vi "Error Handler - Message Handling Loop.vi"(8 "error in (no error)":errorcluster, 10 "Ignore Errors (Runtime)":i32[](array[numeric]), 11 "Message Queue":refnum<queue>) -> (0 "dup error in":errorcluster, 3 "dup Message Queue":refnum<queue>)   [LabVIEW 2017]
doc: "Process an error that occurred in the Message Handling Loop, either by ignoring it, or generating an \"Exit\" message."
uses:
  Message Queue/Message Cluster.ctl
  Message Queue/Message Queue.lvlib
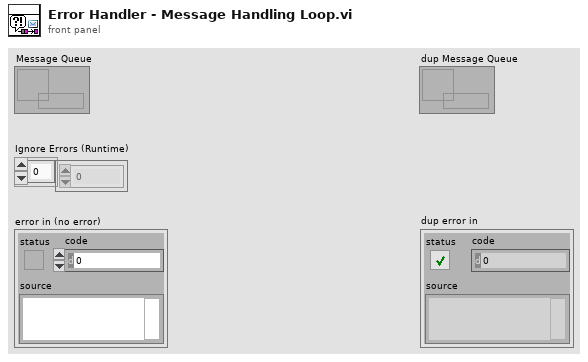
[diagram p1: front panel]
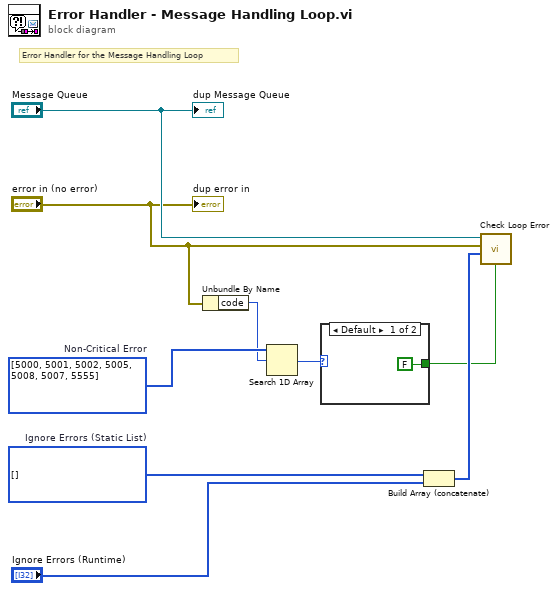
[diagram p0: block diagram]
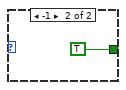
[diagram p2: hidden frame]
diagram:
  w3 = i32[] [5000, 5001, 5002, 5005, 5008, 5007, 5555]  # Non-Critical Error
  w8 = i32[] []  # Ignore Errors (Static List)
  # "Error Handler for the Message Handling Loop"
  n1 = Unbundle By Name("error in (no error)") -> ("code"=w2:i32)
  n2 = Search 1D Array(1D array=w3, element=w2) -> (index of element=w1:i32)  [unwired: 1 in]
  n3 = case shown="Default" w1 {
    tunnel: [FALSE ("Exit on Error? (F)") TRUE ("Exit on Error? (F)")] -> w5
    frame Default {
    }
    frame -1 {
    }
  }
  n4 = Build Array (concatenate)(w8, "Ignore Errors (Runtime)") -> (w7:i32[])
  n5 = call "Check Loop Error.vi"("Exit on Error? (F)"=w5, "Ignore Errors"=w7, "error to process"="error in (no error)", "Message Queue"="Message Queue") -> ()  [unwired: 6 in, 2 out]
  "dup Message Queue" <- "Message Queue"
  "dup error in" <- "error in (no error)"
